vi "Add Item To Tree.vi"(4 "Child Only? (true)":bool=TRUE, 6 "Child Text":string, 7 "TreeControl in":refnum<vi>, 8 "Parent Tag":string, 9 "Child Position":i32, 10 "Left Cell String":string, 11 "Child Tag in":string) -> (1 "Child Text out":string)   [LabVIEW 2020, in "Output Sequencer.lvlib" / "Settings UI.lvclass"]
uses:
  Settings UI.lvclass
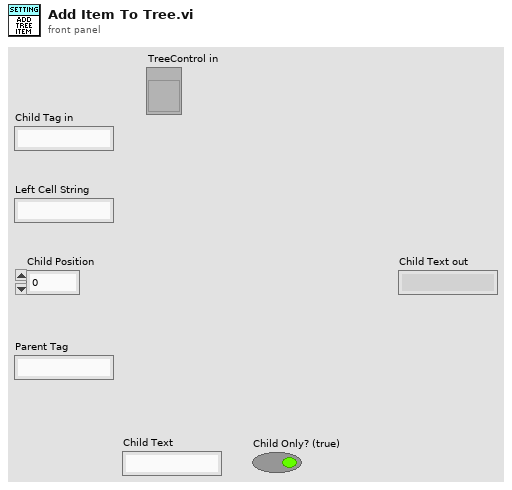
[diagram p1: front panel]
types:
  T1 = typedef "Output Sequencer.lvlib/Settings UI.lvclass/Tree Item Settings.ctl" = cluster{"Tree Label":string, "Indent Level":i32, "Data Type":T2, "Numeric Range":cluster{"Min":dbl, "Max":dbl, "Inc":dbl}, "Allowed Values":string[], "Default Value":string, "Description":string}
  T2 = typedef "Output Sequencer.lvlib/Settings UI.lvclass/Data Type.ctl" = i16
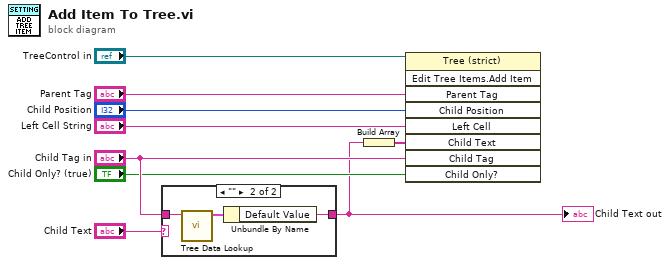
[diagram p0: block diagram]
diagram:
  n1 = case shown="\"\"" "Child Text" {
    selector: "Child Text" -> [w10 _]
    tunnel: "Child Tag in" -> [_ w13]
    tunnel: [w10 w12] -> w2
    frame Default {
    }
    frame "" {
      n2 = call "Tree Data Lookup.vi"("Tag in"=w13) -> ("Tree Data"=w11:T1)  [unwired: 5 in, 5 out]
      n3 = Unbundle By Name(w11) -> ("Default Value"=w12:string)
    }
  }
  "Child Text out" <- w2
  n4 = Build Array(w2) -> (w1:string[])
  n5 = invoke class="Tree (strict)" method="Edit Tree Items.Add Item"(reference="TreeControl in", "Parent Tag"="Parent Tag", "Child Position"="Child Position", "Left Cell"="Left Cell String", "Child Text"=w1, "Child Tag"="Child Tag in", "Child Only?"="Child Only? (true)") -> ()  [unwired: 2 in, 9 out]
